vi "MAIN.vi"() -> ()   [LabVIEW 2015]
uses:
  <vilib>/addons/database/Connection.llb/Conn ObjectReference.ctl
  <vilib>/Utility/miscctls.llb/LVPointTypeDef.ctl
  <vilib>/Utility/file.llb/Read Delimited Spreadsheet (string).vi
  <vilib>/addons/database/Connection.llb/DB Tools Open Connec (Path).vi
  <vilib>/Utility/file.llb/Write Delimited Spreadsheet (string).vi
  <vilib>/addons/database/NI_Database_API.lvlib
panel:
  in  "MATOME":string
  out "userInfo":T1
  out "Connection Database":bool
  out "connection reference":T2
  out "info database":T3
  in  "Update to Database":bool
  out "size(s) 2":i32
  out "size(s)":i32
  out "Status":string
  out "LOT 2":string
  out "LOT 1":string
  out "mau array":string[][](array[string])
  in  "Create file program":bool
  out "sw array":string[][](array[string])
  out "matrix array":string[][](array[string])
  out "ong2 array":string[][](array[string])
  out "ong1 array":string[][](array[string])
  out "jigu array":string[][](array[string])
  in  "File Path Control":path caption="Load File"
  in  "STEP":string
  in  "REV":string
  in  "MODEL":string
  in  "Stop Button":bool
  in  "Save file":bool
  in  "Table Control":string[][](table)
  # "WRITE PROGRAM FOR CONTROL BOX MATOME"
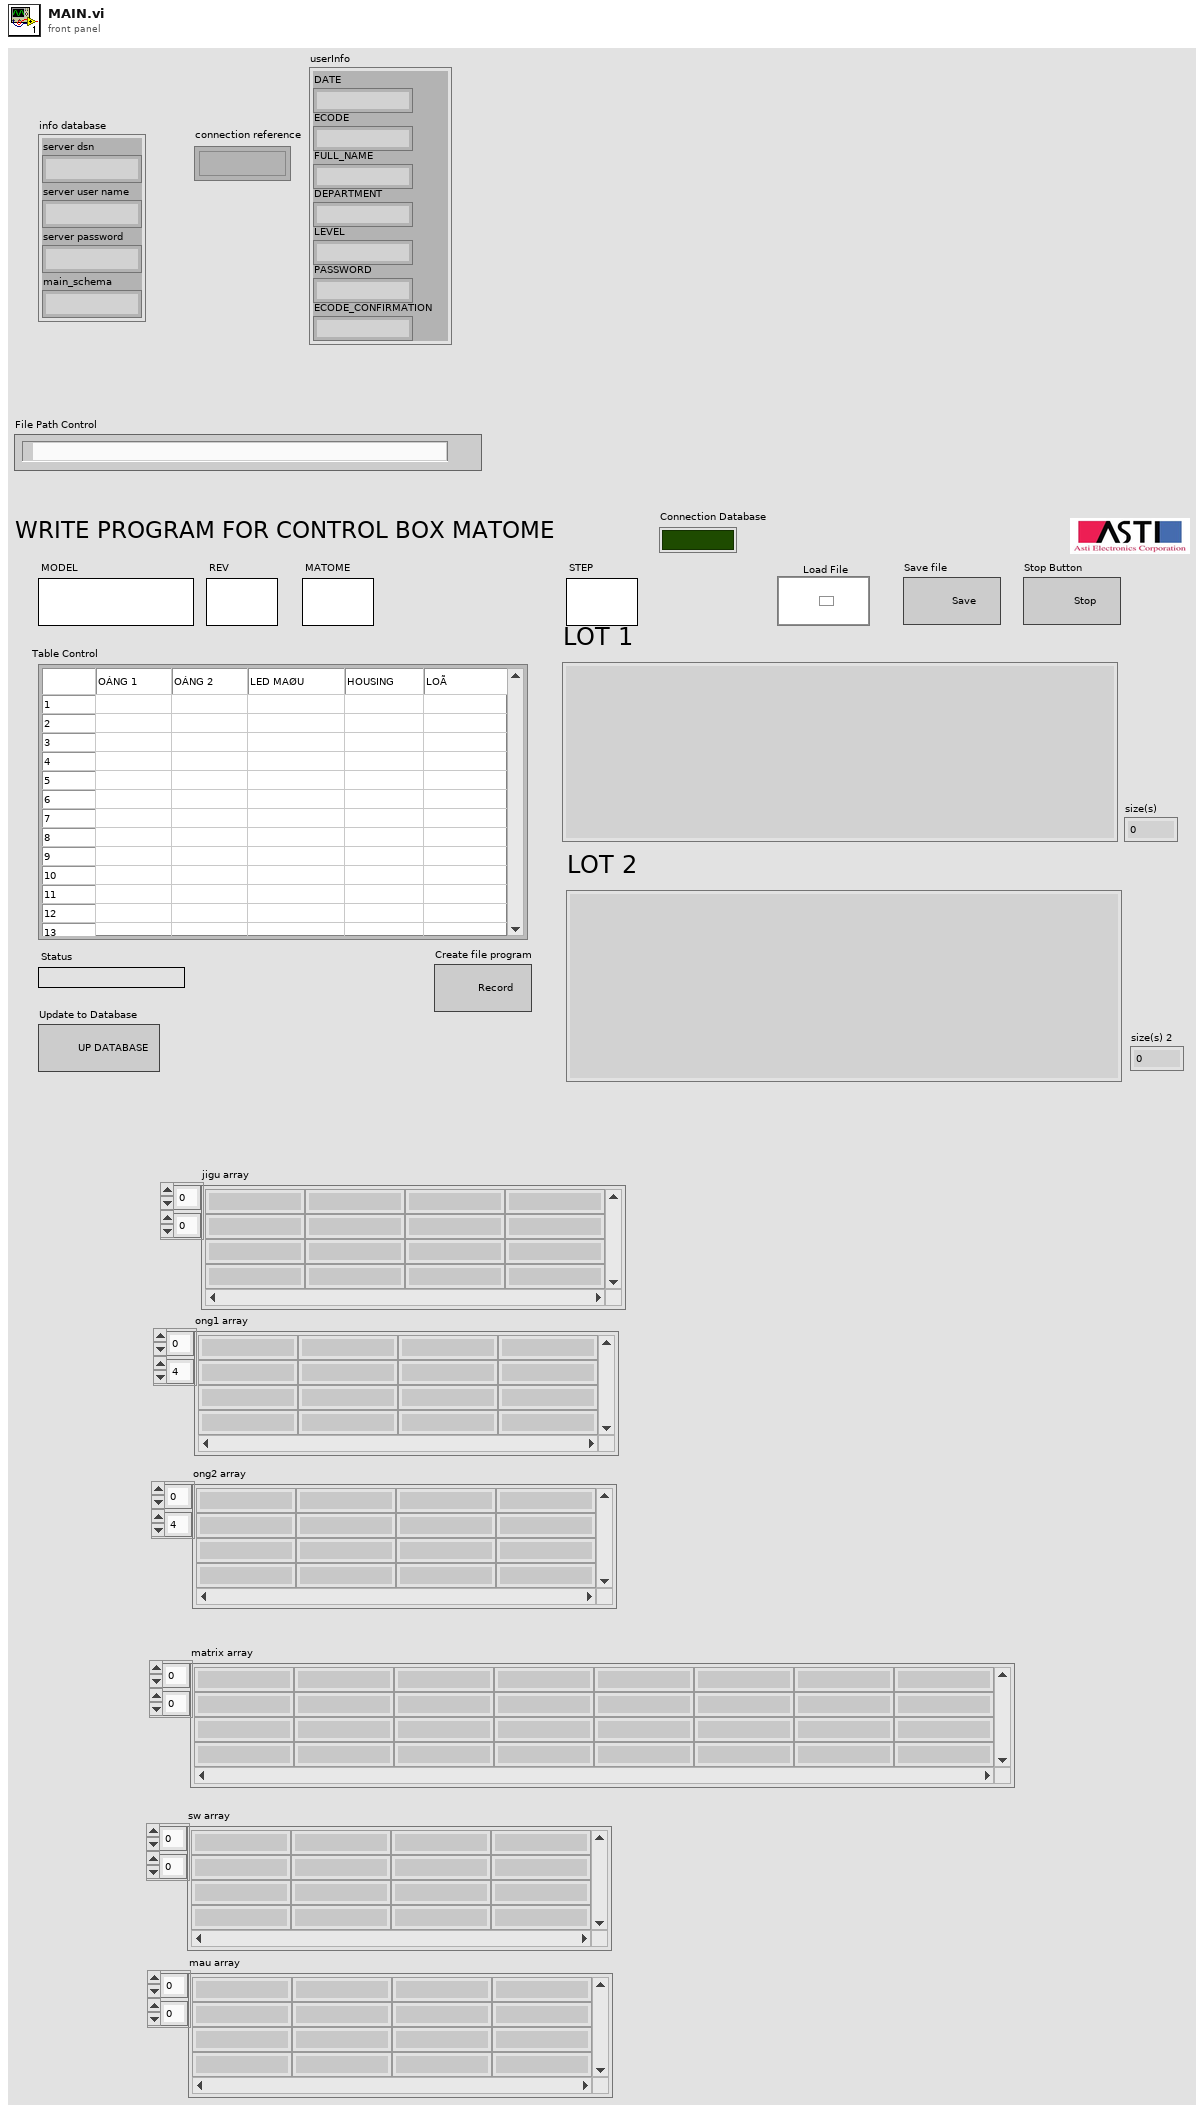
[diagram p1: front panel]
types:
  T1 = cluster{"DATE":string, "ECODE":string, "FULL_NAME":string, "DEPARTMENT":string, "LEVEL":string, "PASSWORD":string, "ECODE_CONFIRMATION":string}
  T2 = typedef "NI_Database_API.lvlib/Conn ObjectReference.ctl" = refnum<k1>
  T3 = cluster{"server dsn":string, "server user name":string, "server password":string, "main_schema":string}
  T4 = typedef "LVPointTypeDef.ctl" = cluster{"Horizontal":i16, "Vertical":i16}
  T5 = cluster{"date/time string":string, "LOT 1":string, "LOT 2":string, "ECODE":string}
  T6 = cluster{"date/time string":string, "MODEL":string, "REV":string, "LOT 1":string, "LOT 2":string, "ECODE":string, "MATOME":string}
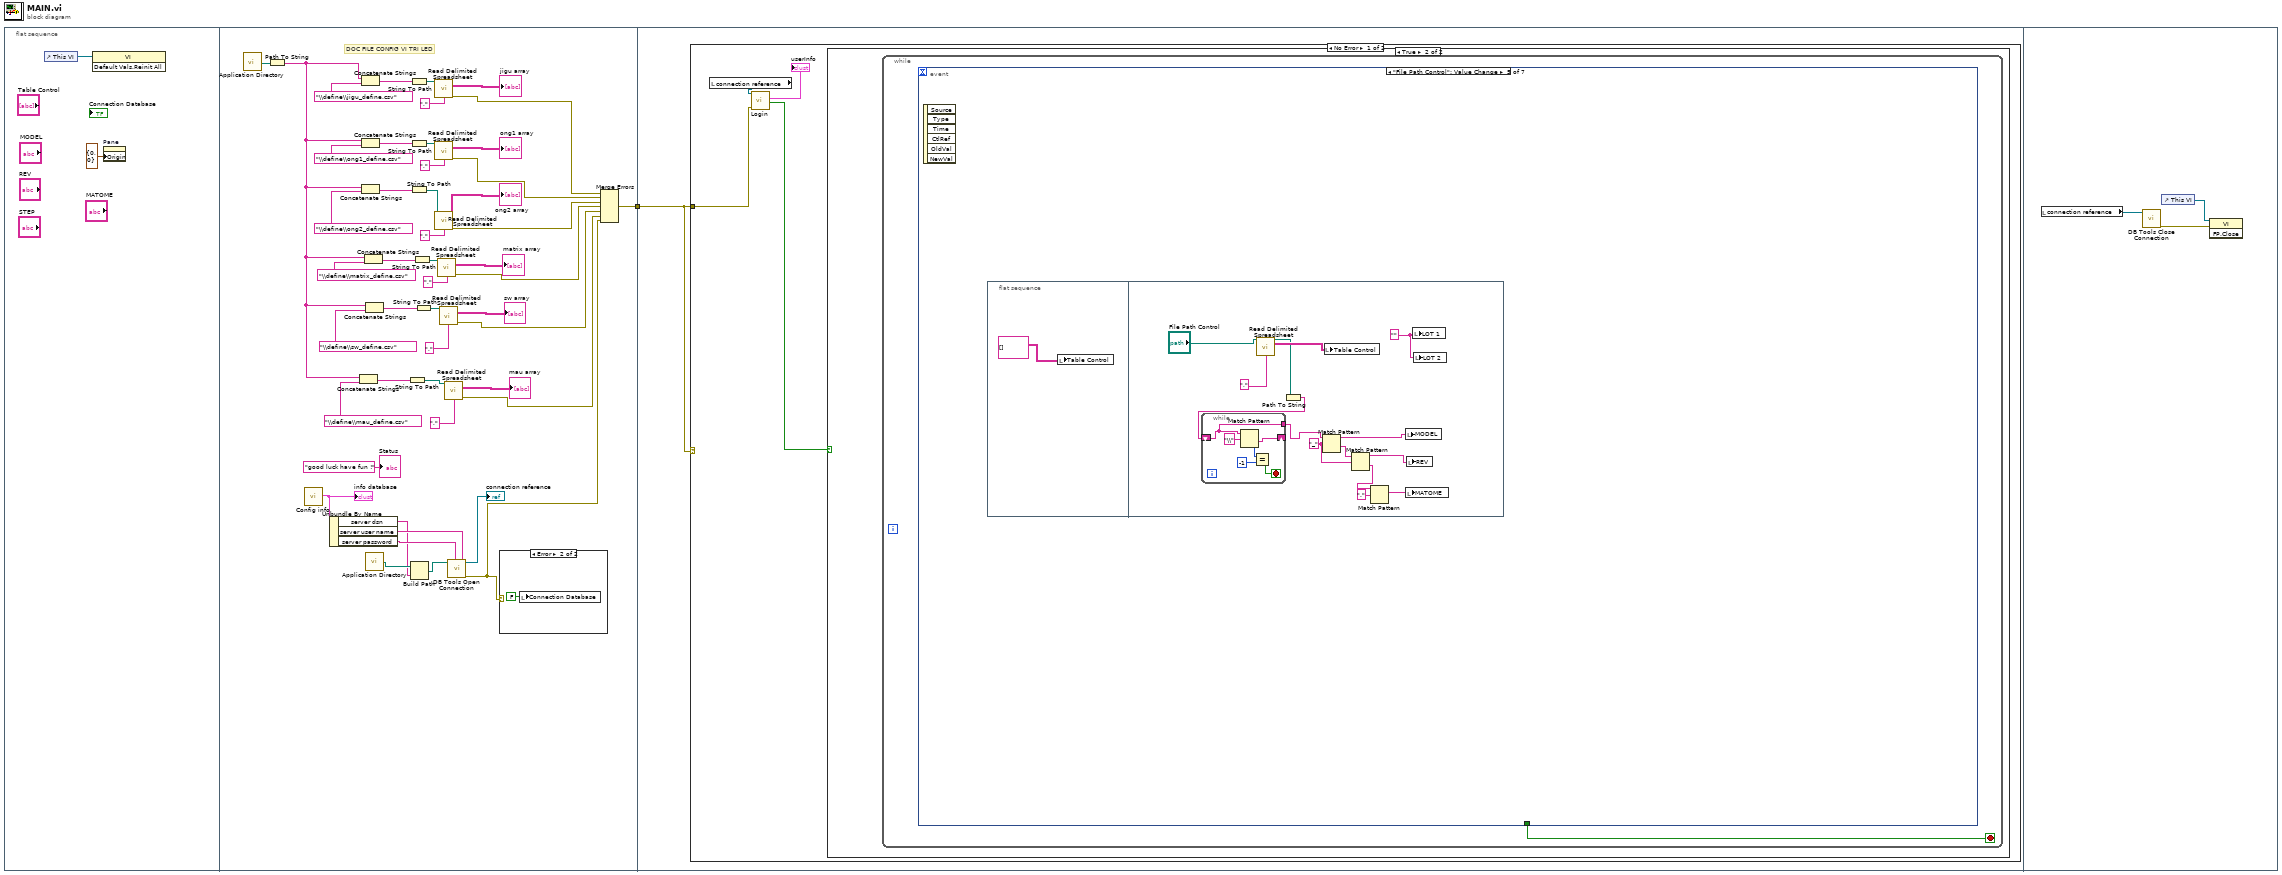
[diagram p0: block diagram]
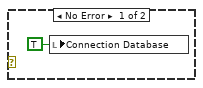
[diagram p2: hidden frame]
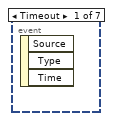
[diagram p4: hidden frame]
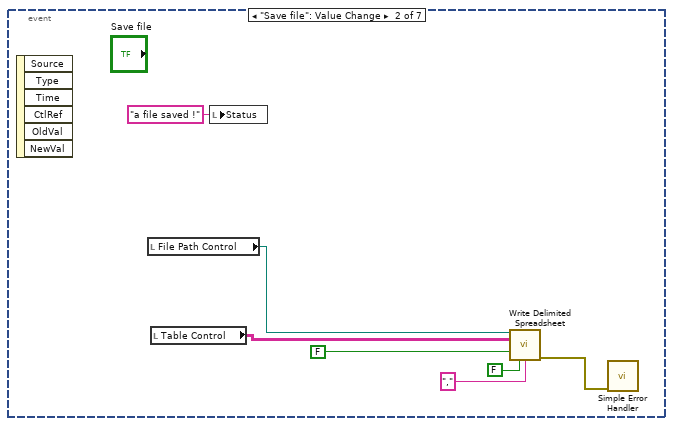
[diagram p5: hidden frame]
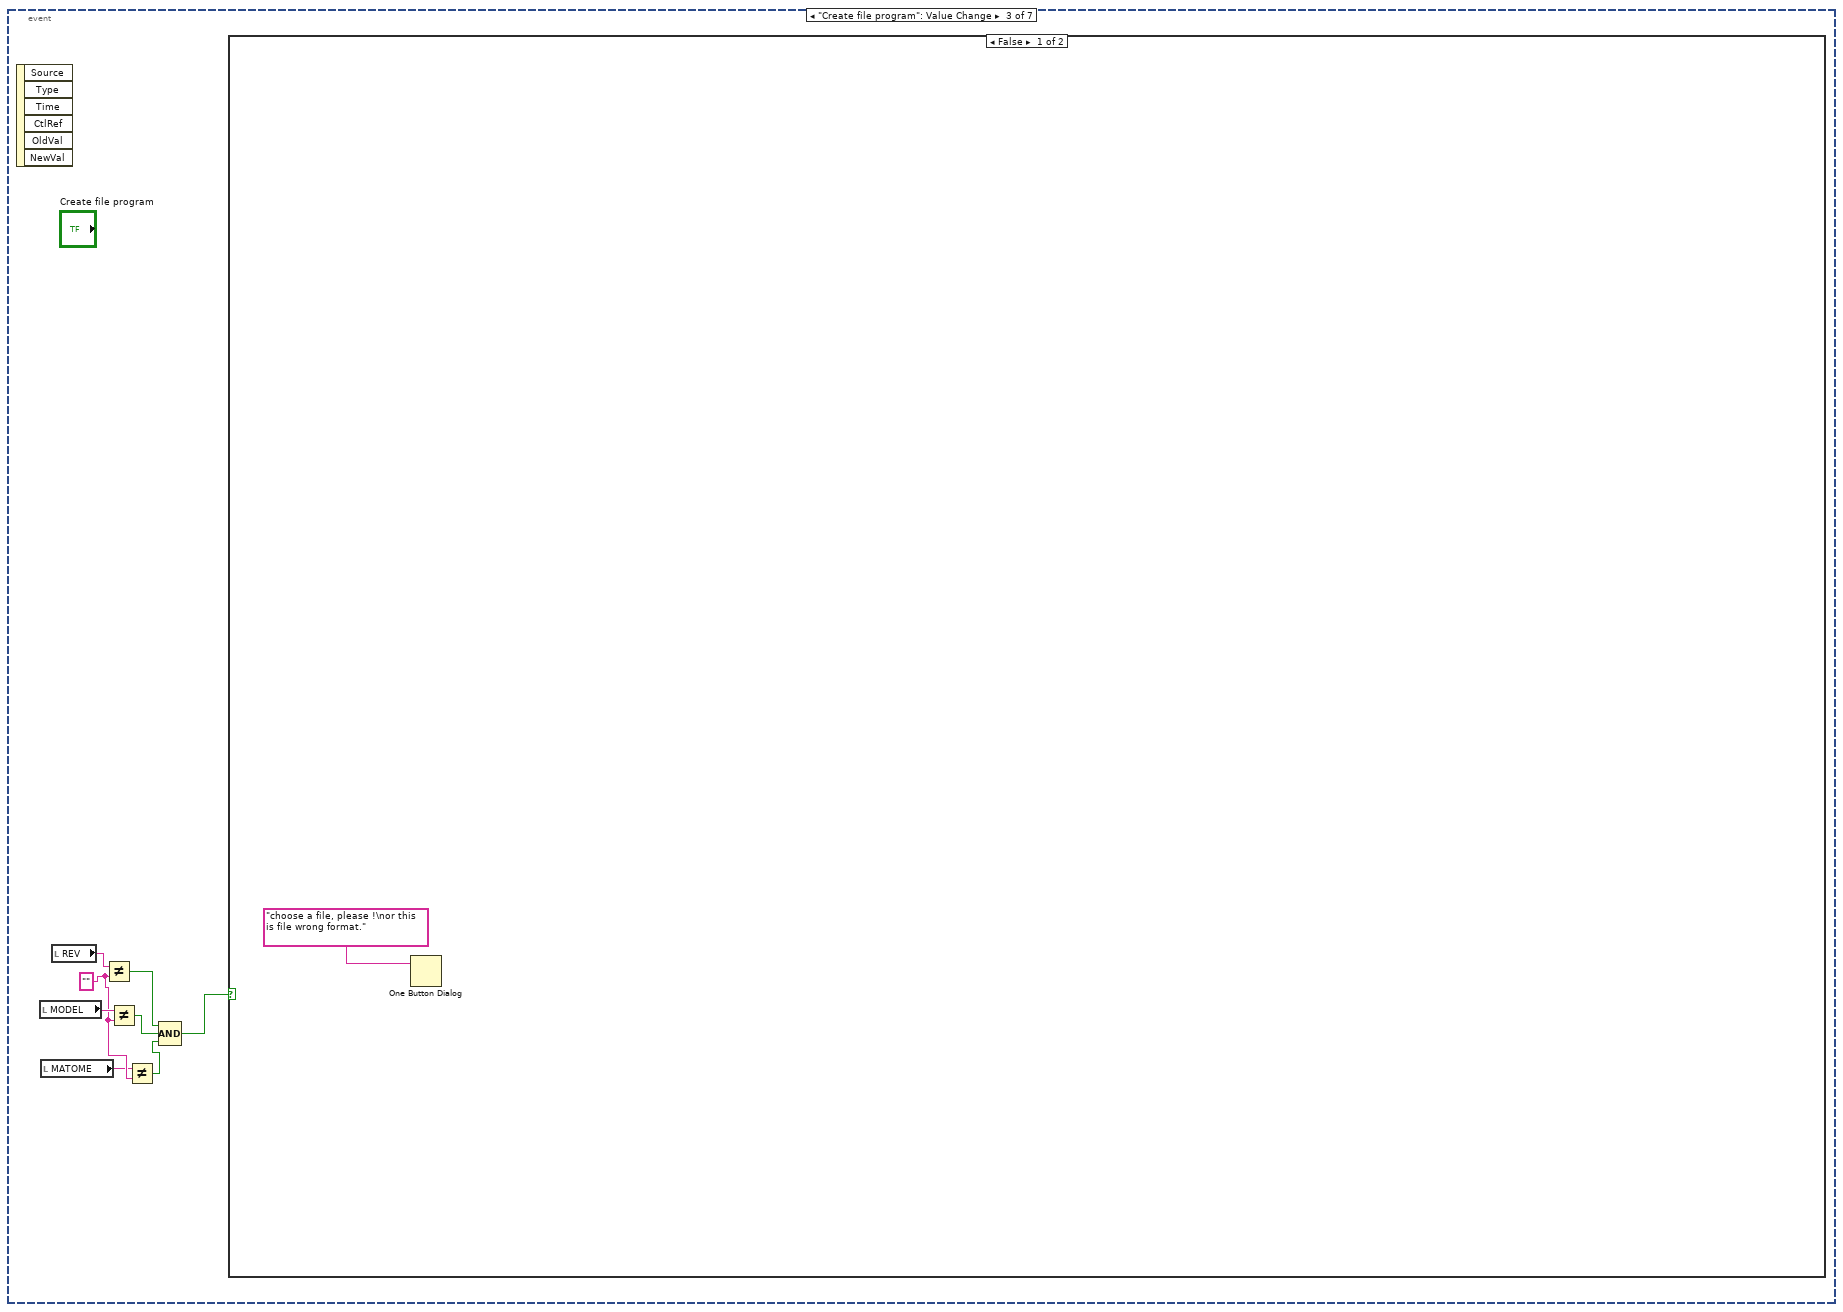
[diagram p6: hidden frame]
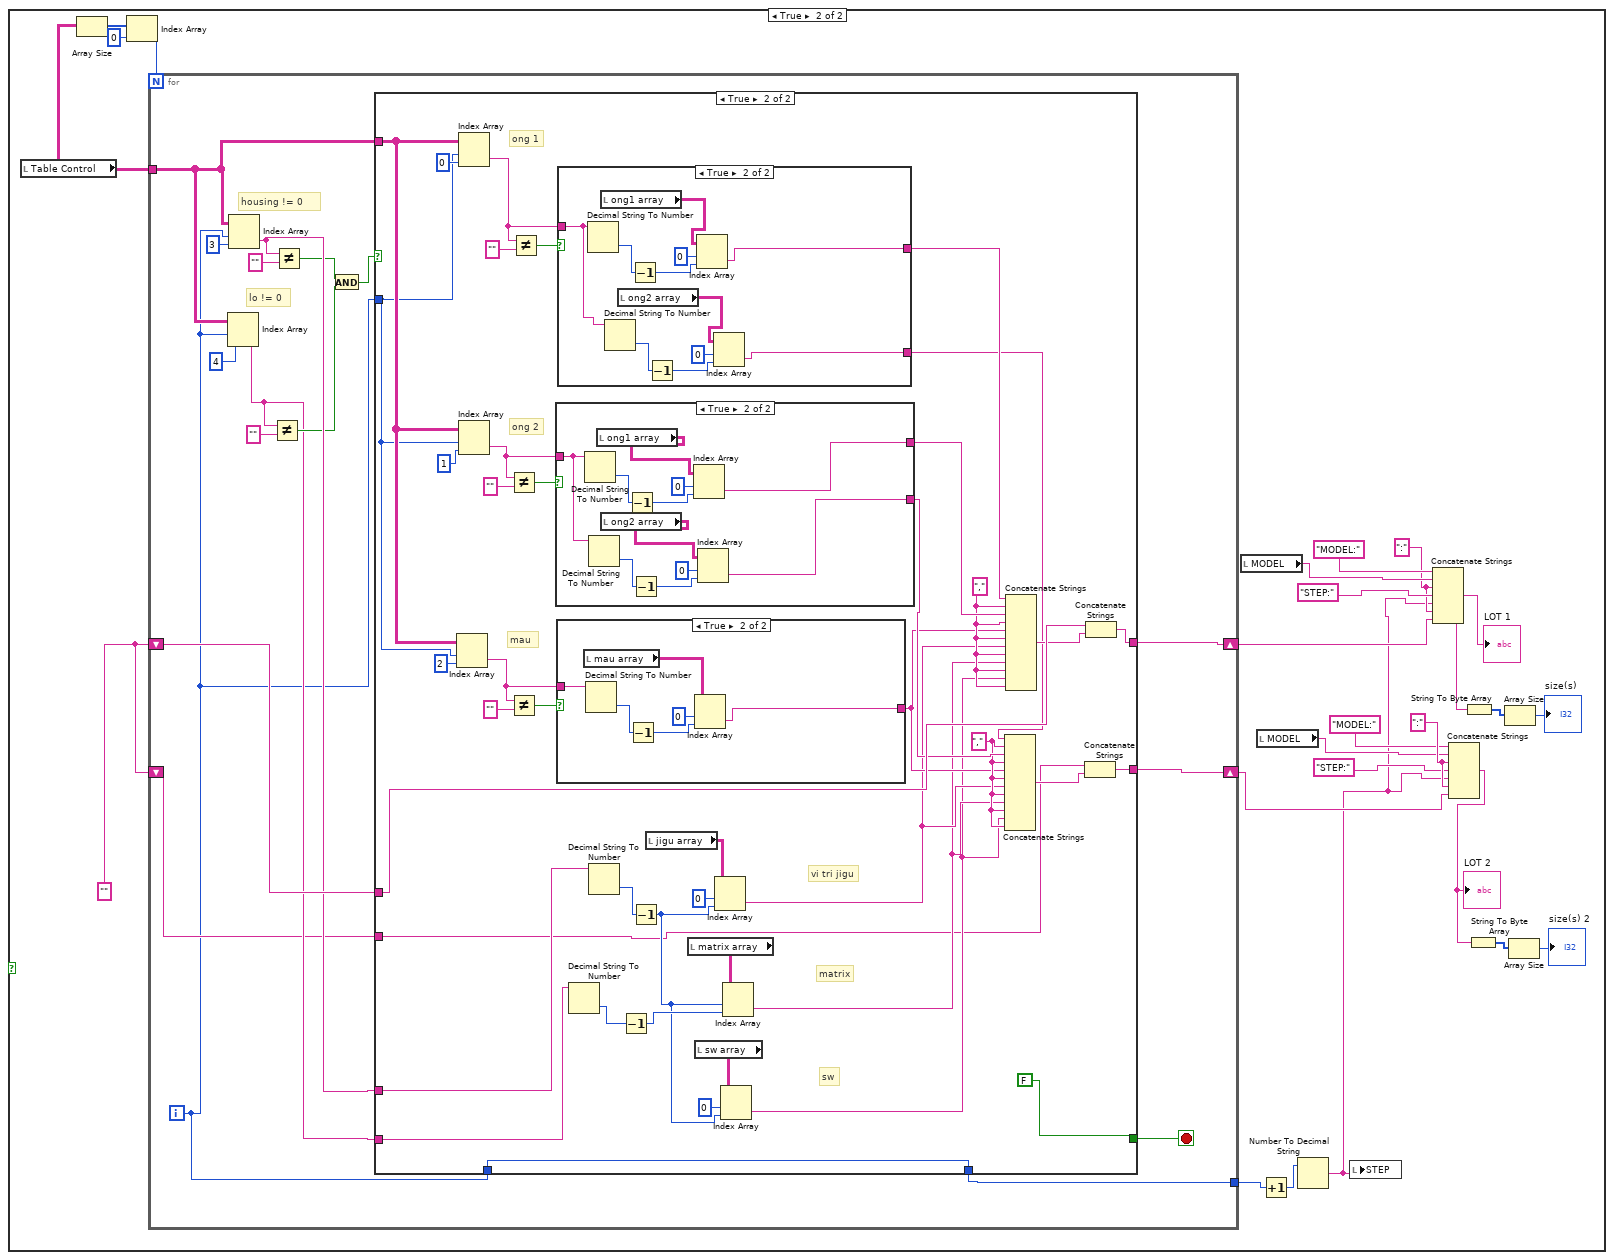
[diagram p7: hidden frame]
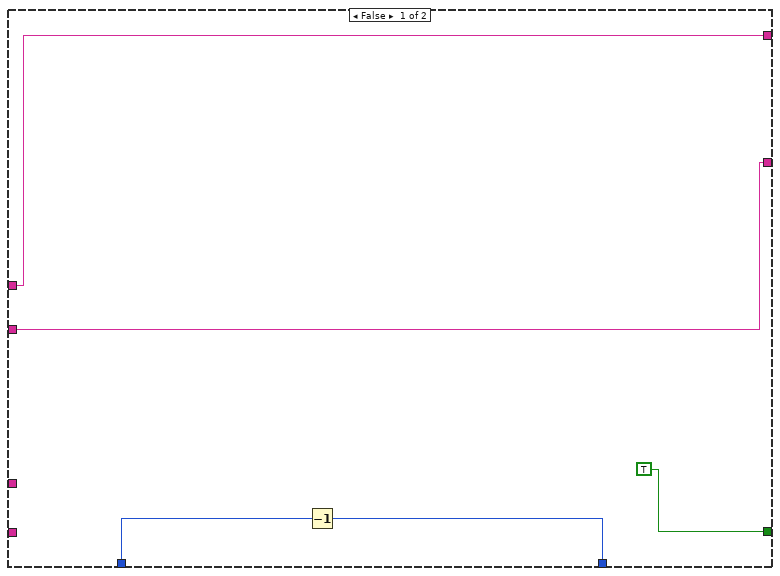
[diagram p8: hidden frame]
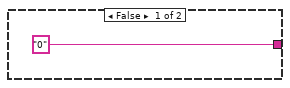
[diagram p9: hidden frame]
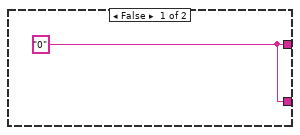
[diagram p10: hidden frame]
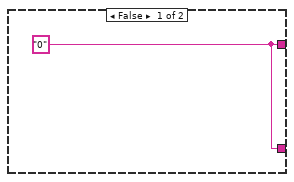
[diagram p11: hidden frame]
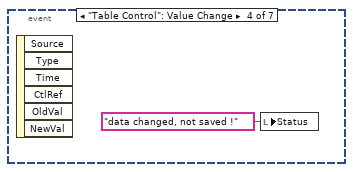
[diagram p12: hidden frame]
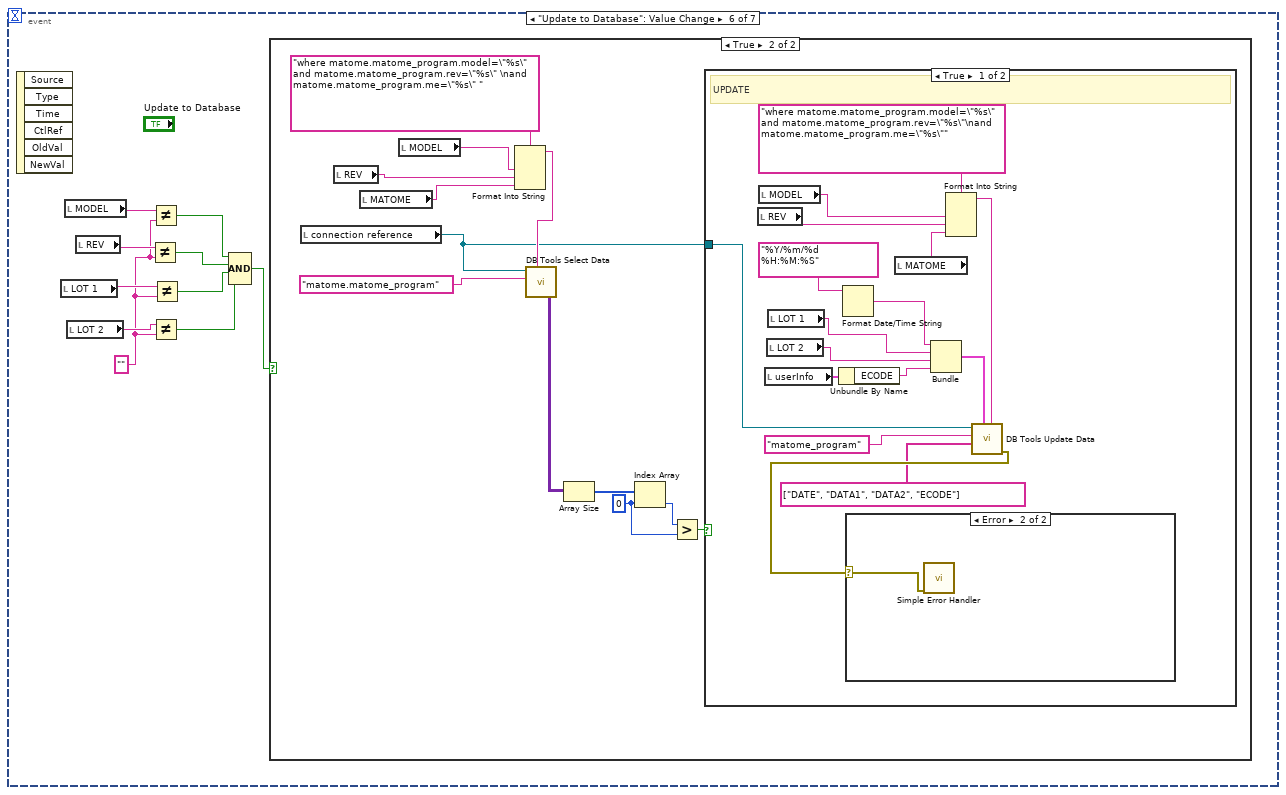
[diagram p13: hidden frame]
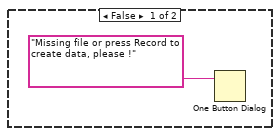
[diagram p14: hidden frame]
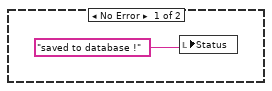
[diagram p15: hidden frame]
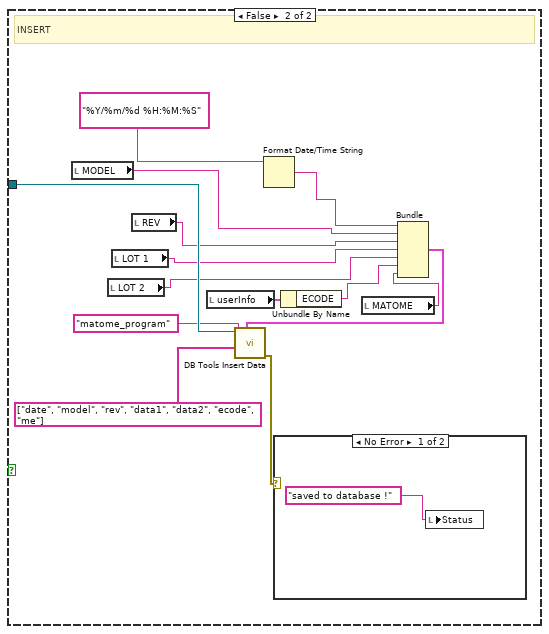
[diagram p16: hidden frame]
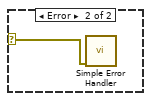
[diagram p17: hidden frame]
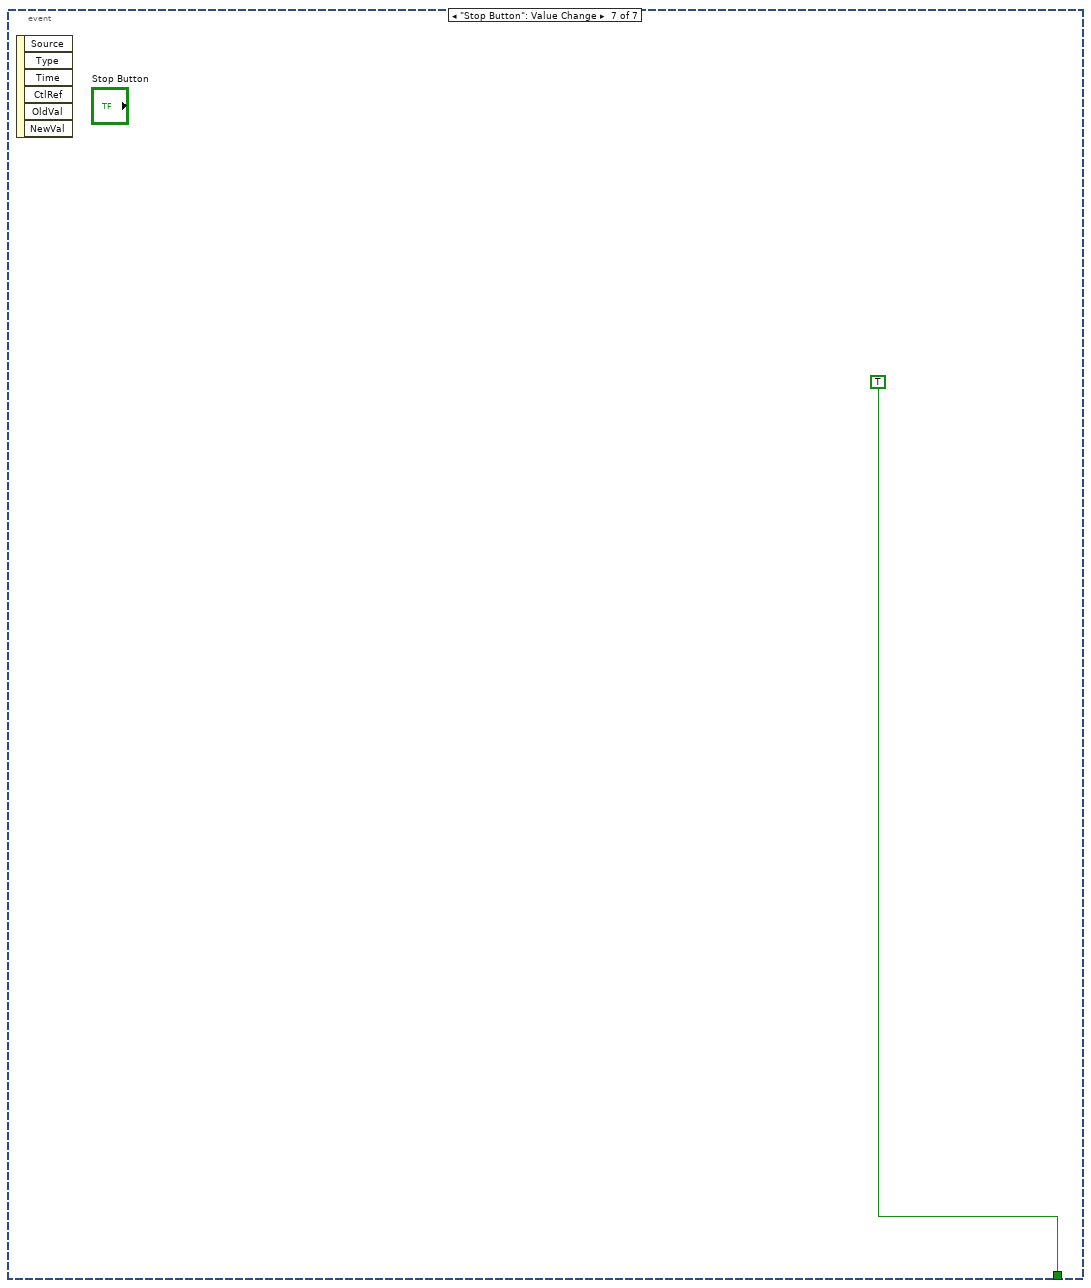
[diagram p18: hidden frame]
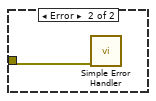
[diagram p19: hidden frame]
diagram:
  n1 = flat-sequence {
    tunnel: [w4] -> w1
    tunnel: w1 -> [w54]
    frame #0 {
      n2 = control-ref of="This VI"() -> (w3:refnum<vi>)
      n3 = invoke class="VI" method="Default Vals.Reinit All"(reference=w3) -> ()  [unwired: 2 in, 3 out]
      n4 = property on="Pane" class="Pane"("Origin"=T4 {"Horizontal"=0, "Vertical"=0}) -> ()  [unwired: 2 in, 2 out]
    }
    frame #1 {
      # "DOC FILE CONFIG VI TRI LED"
      n5 = call <vilib>:"Application Directory.vi"() -> ("Application Directory"=w51:path)
      n6 = Path To String(path=w51) -> (string=w20:string)
      n7 = call "Config info.vi"() -> ("info database"=w18:T3)  [unwired: 10 in, 1 out]
      "info database" <- w18
      n8 = Unbundle By Name(w18) -> ("server dsn"=w14:string, "server user name"=w17:string, "server password"=w16:string)
      n9 = Concatenate Strings(w20, "\\define\\mau_define.csv" ("string")) -> (w22:string)
      n10 = Concatenate Strings(w20, "\\define\\jigu_define.csv" ("string")) -> (w49:string)
      n11 = Concatenate Strings(w20, "\\define\\ong1_define.csv" ("string")) -> (w42:string)
      n12 = Concatenate Strings(w20, "\\define\\ong2_define.csv" ("string")) -> (w39:string)
      n13 = Concatenate Strings(w20, "\\define\\matrix_define.csv" ("string")) -> (w32:string)
      n14 = Concatenate Strings(w20, "\\define\\sw_define.csv" ("string")) -> (w29:string)
      n15 = call <vilib>:"Application Directory.vi"() -> ("Application Directory"=w15:path)
      n16 = String To Path(string=w22) -> (path=w23:path)
      n17 = Build Path(base path=w15, name or relative path=w14) -> (appended path=w13:path)
      n18 = String To Path(string=w49) -> (path=w48:path)
      n19 = String To Path(string=w42) -> (path=w43:path)
      n20 = String To Path(string=w39) -> (path=w38:path)
      n21 = String To Path(string=w32) -> (path=w33:path)
      n22 = String To Path(string=w29) -> (path=w28:path)
      n23 = call-poly <vilib>:"Read Delimited Spreadsheet.vi"("file path (dialog if empty)"=w48, "delimiter (\\t)"="," ("delimiter (\\t)")) -> ("all rows"=→"jigu array":string[][], "error out"=w11:errorcluster)  [unwired: 8 in, 4 out]
      n24 = call-poly <vilib>:"Read Delimited Spreadsheet.vi"("file path (dialog if empty)"=w43, "delimiter (\\t)"="," ("delimiter (\\t)")) -> ("all rows"=→"ong1 array":string[][], "error out"=w10:errorcluster)  [unwired: 8 in, 4 out]
      n25 = call-poly <vilib>:"Read Delimited Spreadsheet.vi"("file path (dialog if empty)"=w38, "delimiter (\\t)"="," ("delimiter (\\t)")) -> ("all rows"=→"ong2 array":string[][], "error out"=w9:errorcluster)  [unwired: 8 in, 4 out]
      n26 = call-poly <vilib>:"Read Delimited Spreadsheet.vi"("file path (dialog if empty)"=w33, "delimiter (\\t)"="," ("delimiter (\\t)")) -> ("all rows"=→"matrix array":string[][], "error out"=w8:errorcluster)  [unwired: 8 in, 4 out]
      n27 = call-poly <vilib>:"Read Delimited Spreadsheet.vi"("file path (dialog if empty)"=w28, "delimiter (\\t)"="," ("delimiter (\\t)")) -> ("all rows"=→"sw array":string[][], "error out"=w7:errorcluster)  [unwired: 8 in, 4 out]
      n28 = call-poly <vilib>:"Read Delimited Spreadsheet.vi"("file path (dialog if empty)"=w23, "delimiter (\\t)"="," ("delimiter (\\t)")) -> ("all rows"=→"mau array":string[][], "error out"=w6:errorcluster)  [unwired: 8 in, 4 out]
      n29 = call-poly <vilib>:"DB Tools Open Connection.vi"("password"=w16, "userID"=w17, "connection information"=w13) -> ("error out"=w5:errorcluster, "connection reference"=→"connection reference":T2)  [unwired: 5 in]
      n30 = case shown="Error" w5 {
        frame No Error {
          n31 = local write "Connection Database"(TRUE ("Connection Database")) -> ()
        }
        frame Error {
          n32 = local write "Connection Database"(FALSE ("Connection Database")) -> ()
        }
      }
      n33 = Merge Errors(w11, w10, w9, w8, w7, w6, w5) -> (w4:errorcluster)
      "Status" <- "good luck have fun !" ("Status")
    }
    frame #2 {
      n34 = case shown="No Error" w54 {
        tunnel: w54 -> [w55 w276]
        frame No Error {
          n35 = local read "connection reference"() -> (w58:T2)
          n36 = call "Login.vi"("error in (no error)"=w55, "connection reference"=w58) -> ("valid?"=w57:bool, "userInfo"=→"userInfo":T1)  [unwired: 6 in, 2 out]
          n37 = case shown="True" w57 {
            frame False {
            }
            frame True {
              n38 = while {
                stop <- w59 stop-if-true
                n39 = event shown="[4] \"File Path Control\": Value Change" {
                  selector: _ -> [_ _ _ _ _ _ _]
                  dyn-events: _ -> [_ _ _ _ _ _ _]
                  timeout: _ -> [_ _ _ _ _ _ _]
                  tunnel: [_ _ _ _ _ _ TRUE] -> w59
                  event Timeout {
                    n40 = event-data() -> ()  [unwired: 1 in, 3 out]
                  }
                  event "Save file": Value Change {
                    n41 = event-data() -> ()  [unwired: 1 in, 6 out]
                    n42 = local read "File Path Control"() -> (w66:path)
                    n43 = local read "Table Control"() -> (w65:string[][])
                    n44 = local write "Status"("a file saved !" ("Status")) -> ()
                    n45 = call-poly <vilib>:"Write Delimited Spreadsheet.vi"("file path (dialog if empty)"=w66, "2D data"=w65, "append to file? (F)"=FALSE, "transpose? (F)"=FALSE, "delimiter (\\t)"="," ("delimiter (\\t)")) -> ("error out"=w61:errorcluster)  [unwired: 9 in, 1 out]
                    n46 = call <vilib>:"Simple Error Handler.vi"("error in (no error)"=w61) -> ()  [unwired: 4 in, 5 out]
                  }
                  event "Create file program": Value Change {
                    w72 = ""
                    n47 = event-data() -> ()  [unwired: 1 in, 6 out]
                    n48 = local read "MODEL"() -> (w73:string)
                    n49 = local read "MATOME"() -> (w71:string)
                    n50 = local read "REV"() -> (w74:string)
                    n51 = Not Equal?(x=w74, y=w72) -> (x != y?=w70:bool)
                    n52 = Not Equal?(x=w73, y=w72) -> (x != y?=w69:bool)
                    n53 = Not Equal?(x=w71, y=w72) -> (x != y?=w68:bool)
                    n54 = Compound Arithmetic op=AND(w70, w69, w68) -> (w67:bool)
                    n55 = case shown="False" w67 {
                      frame False {
                        n56 = One Button Dialog(message="choose a file, please !\nor this is file wrong format.") -> ()  [unwired: 1 in, 1 out]
                      }
                      frame True {
                        w89 = ":" ("string")
                        w91 = ":" ("string")
                        w95 = ""
                        n57 = local read "Table Control"() -> (w96:string[][])
                        n58 = Array Size(array=w96) -> (size(s)=w99:i32[])
                        n59 = Index Array(array=w99, index=0) -> (element=w97:i32)
                        n60 = for {
                          N: w97 -> [_]
                          tunnel: w96 -> [w110]
                          shift-right: [w105] -> w90
                          shift-left: w95 -> [w114]
                          shift-right: [w103] -> w86
                          shift-left: w95 -> [w102]
                          tunnel: [w100] -> w84
                          i -> [w101]
                          stop <- w104 stop-if-true
                          # "lo != 0"
                          # "housing != 0"
                          n61 = Index Array(array=w110, index (row)=w101, index (col)=4 ("disabled index (col)")) -> (element=w106:string)
                          n62 = Index Array(array=w110, index (row)=w101, index (col)=3 ("disabled index (col)")) -> (element=w113:string)
                          n63 = Not Equal?(x=w106, y="") -> (x != y?=w108:bool)
                          n64 = Not Equal?(x=w113, y="") -> (x != y?=w109:bool)
                          n65 = And(x=w109, y=w108) -> (x .and. y?=w107:bool)
                          n66 = case shown="True" w107 {
                            tunnel: w114 -> [w121 w136]
                            tunnel: w110 -> [_ w152]
                            tunnel: w101 -> [_ w151]
                            tunnel: w113 -> [_ w147]
                            tunnel: w106 -> [_ w145]
                            tunnel: [w121 w134] -> w105
                            tunnel: [TRUE FALSE] -> w104
                            tunnel: [w119 w124] -> w103
                            tunnel: w102 -> [w119 w123]
                            tunnel: w101 -> [w118 w122]
                            tunnel: [w117 w122] -> w100
                            frame False {
                              n67 = Decrement(x=w118) -> (x-1=w117:i32)
                            }
                            frame True {
                              w129 = ","
                              w137 = ","
                              # "sw"
                              # "matrix"
                              # "vi tri jigu"
                              # "mau"
                              # "ong 2"
                              # "ong 1"
                              n68 = Index Array(array=w152, index (row)=w151, index (col)=2 ("disabled index (col)")) -> (element=w153:string)
                              n69 = Index Array(array=w152, index (row)=w151, index (col)=0 ("disabled index (col)")) -> (element=w161:string)
                              n70 = Index Array(array=w152, index (row)=w151, index (col)=1 ("disabled index (col)")) -> (element=w160:string)
                              n71 = Not Equal?(x=w160, y="") -> (x != y?=w159:bool)
                              n72 = Not Equal?(x=w153, y="") -> (x != y?=w154:bool)
                              n73 = Not Equal?(x=w161, y="") -> (x != y?=w162:bool)
                              n74 = case shown="True" w159 {
                                tunnel: [w172 w180] -> w138
                                tunnel: w160 -> [_ w174]
                                tunnel: [w172 w173] -> w130
                                frame False {
                                w172 = "0"
                                }
                                frame True {
                                n75 = Decimal String To Number(string=w174) -> (number=w182:i32)  [unwired: 2 in, 1 out]
                                n76 = Decimal String To Number(string=w174) -> (number=w176:i32)  [unwired: 2 in, 1 out]
                                n77 = local read "ong1 array"() -> (w179:string[][])
                                n78 = local read "ong2 array"() -> (w178:string[][])
                                n79 = Decrement(x=w182) -> (x-1=w181:i32)
                                n80 = Decrement(x=w176) -> (x-1=w177:i32)
                                n81 = Index Array(array=w179, index (row)=0, index (col)=w181) -> (element=w180:string)
                                n82 = Index Array(array=w178, index (row)=0, index (col)=w177) -> (element=w173:string)
                                }
                              }
                              n83 = case shown="True" w154 {
                                tunnel: ["0" w166] -> w128
                                tunnel: w153 -> [_ w169]
                                frame False {
                                }
                                frame True {
                                n84 = local read "mau array"() -> (w171:string[][])
                                n85 = Decimal String To Number(string=w169) -> (number=w168:i32)  [unwired: 2 in, 1 out]
                                n86 = Decrement(x=w168) -> (x-1=w167:i32)
                                n87 = Index Array(array=w171, index (row)=0, index (col)=w167) -> (element=w166:string)
                                }
                              }
                              n88 = case shown="True" w162 {
                                tunnel: [w184 w192] -> w139
                                tunnel: w161 -> [_ w186]
                                tunnel: [w184 w185] -> w131
                                frame False {
                                w184 = "0"
                                }
                                frame True {
                                n89 = Decimal String To Number(string=w186) -> (number=w194:i32)  [unwired: 2 in, 1 out]
                                n90 = local read "ong1 array"() -> (w191:string[][])
                                n91 = Decimal String To Number(string=w186) -> (number=w188:i32)  [unwired: 2 in, 1 out]
                                n92 = local read "ong2 array"() -> (w190:string[][])
                                n93 = Decrement(x=w194) -> (x-1=w193:i32)
                                n94 = Decrement(x=w188) -> (x-1=w189:i32)
                                n95 = Index Array(array=w191, index (row)=0, index (col)=w193) -> (element=w192:string)
                                n96 = Index Array(array=w190, index (row)=0, index (col)=w189) -> (element=w185:string)
                                }
                              }
                              n97 = Decimal String To Number(string=w145) -> (number=w144:i32)  [unwired: 2 in, 1 out]
                              n98 = Decimal String To Number(string=w147) -> (number=w148:i32)  [unwired: 2 in, 1 out]
                              n99 = Decrement(x=w144) -> (x-1=w143:i32)
                              n100 = Decrement(x=w148) -> (x-1=w141:i32)
                              n101 = local read "jigu array"() -> (w150:string[][])
                              n102 = local read "matrix array"() -> (w146:string[][])
                              n103 = local read "sw array"() -> (w142:string[][])
                              n104 = Index Array(array=w150, index (row)=0, index (col)=w141) -> (element=w127:string)
                              n105 = Index Array(array=w142, index (row)=0 ("disabled index (row)"), index (col)=w141) -> (element=w125:string)
                              n106 = Index Array(array=w146, index (row)=w141, index (col)=w143) -> (element=w126:string)
                              n107 = Concatenate Strings(w131, w129, w130, w129, w128, w129, w127, w129, w126, w129, w125, w129) -> (w132:string)
                              n108 = Concatenate Strings(w139, w137, w138, w137, w128, w137, w127, w137, w126, w137, w125, w137) -> (w135:string)
                              n109 = Concatenate Strings(w123, w132) -> (w124:string)
                              n110 = Concatenate Strings(w136, w135) -> (w134:string)
                            }
                          }
                        }
                        n111 = local read "MODEL"() -> (w93:string)
                        n112 = local read "MODEL"() -> (w88:string)
                        n113 = Increment(x=w84) -> (x+1=w85:i32)
                        n114 = Number To Decimal String(number=w85) -> (decimal integer string=w82:string)  [unwired: 1 in]
                        n115 = local write "STEP"(w82) -> ()
                        n116 = Concatenate Strings("MODEL:" ("string"), w93, w91, "STEP:" ("string"), w82, w91, w90) -> (w81:string)
                        "LOT 1" <- w81
                        n117 = Concatenate Strings("MODEL:" ("string"), w88, w89, "STEP:" ("string"), w82, w89, w86) -> (w76:string)
                        "LOT 2" <- w76
                        n118 = String To Byte Array(string=w81) -> (unsigned byte array=w80:u8[])
                        n119 = String To Byte Array(string=w76) -> (unsigned byte array=w77:u8[])
                        n120 = Array Size(array=w80) -> (size(s)=→"size(s)":i32)
                        n121 = Array Size(array=w77) -> (size(s)=→"size(s) 2":i32)
                      }
                    }
                  }
                  event "Table Control": Value Change {
                    n122 = event-data() -> ()  [unwired: 1 in, 6 out]
                    n123 = local write "Status"("data changed, not saved !" ("Status")) -> ()
                  }
                  event "File Path Control": Value Change {
                    n124 = event-data() -> ()  [unwired: 1 in, 6 out]
                    n125 = flat-sequence {
                      frame #0 {
                        n126 = local write "Table Control"(string[][] []) -> ()
                      }
                      frame #1 {
                        w198 = ""
                        w202 = "_" ("regular expression")
                        n127 = call-poly <vilib>:"Read Delimited Spreadsheet.vi"("file path (dialog if empty)"="File Path Control", "delimiter (\\t)"="," ("delimiter (\\t)")) -> ("new file path (Not A Path if cancelled)"=w208:path, "all rows"=w209:string[][])  [unwired: 8 in, 4 out]
                        n128 = Path To String(path=w208) -> (string=w207:string)
                        n129 = while {
                          shift-right: [w213] -> _
                          shift-left: w207 -> [w212]
                          tunnel: [w212] -> w206
                          stop <- w214 stop-if-true
                          n130 = Match Pattern(string=w212, regular expression="\\") -> (after substring=w213:string, offset past match=w216:i32)  [unwired: 1 in, 2 out]
                          n131 = Equal?(x=w216, y=-1) -> (x = y?=w214:bool)
                        }
                        n132 = Match Pattern(string=w206, regular expression=w202) -> (before substring=w205:string, after substring=w203:string)  [unwired: 1 in, 2 out]
                        n133 = local write "Table Control"(w209) -> ()
                        n134 = Match Pattern(string=w203, regular expression=w202) -> (before substring=w200:string, after substring=w201:string)  [unwired: 1 in, 2 out]
                        n135 = Match Pattern(string=w201, regular expression=".") -> (match substring=w199:string)  [unwired: 1 in, 3 out]
                        n136 = local write "MODEL"(w205) -> ()
                        n137 = local write "MATOME"(w199) -> ()
                        n138 = local write "REV"(w200) -> ()
                        n139 = local write "LOT 1"(w198) -> ()
                        n140 = local write "LOT 2"(w198) -> ()
                      }
                    }
                  }
                  event "Update to Database": Value Change {
                    w223 = ""
                    n141 = event-data() -> ()  [unwired: 1 in, 6 out]
                    n142 = local read "LOT 1"() -> (w225:string)
                    n143 = local read "MODEL"() -> (w227:string)
                    n144 = local read "LOT 2"() -> (w224:string)
                    n145 = local read "REV"() -> (w226:string)
                    n146 = Not Equal?(x=w226, y=w223) -> (x != y?=w221:bool)
                    n147 = Not Equal?(x=w227, y=w223) -> (x != y?=w222:bool)
                    n148 = Not Equal?(x=w224, y=w223) -> (x != y?=w219:bool)
                    n149 = Not Equal?(x=w225, y=w223) -> (x != y?=w220:bool)
                    n150 = Compound Arithmetic op=AND(w222, w221, w220, w219) -> (w218:bool)
                    n151 = case shown="True" w218 {
                      frame False {
                        n152 = One Button Dialog(message="Missing file or press Record to create data, please !") -> ()  [unwired: 1 in, 1 out]
                      }
                      frame True {
                        w236 = 0 ("index")
                        n153 = local read "connection reference"() -> (w231:T2)
                        n154 = local read "REV"() -> (w230:string)
                        n155 = local read "MATOME"() -> (w229:string)
                        n156 = local read "MODEL"() -> (w232:string)
                        n157 = Format Into String(format string="where matome.matome_program.model=\"%s\" and matome.matome_program.rev=\"%s\" \nand matome.matome_program.me=\"%s\" " ("condition"), w232, w230, w229) -> (resulting string=w233:string)  [unwired: 2 in, 1 out]
                        n158 = call <vilib>:"DB Tools Select Data.vi"("condition"=w233, "table"="matome.matome_program", "connection reference"=w231) -> ("data"=w239:variant[][])  [unwired: 3 in, 2 out]
                        n159 = Array Size(array=w239) -> (size(s)=w238:i32[])
                        n160 = Index Array(array=w238, index=w236) -> (element=w237:i32)
                        n161 = Greater?(x=w237, y=w236) -> (0:w235:bool)
                        n162 = case shown="True" w235 {
                          tunnel: w231 -> [w256 w272]
                          frame True {
                            # "UPDATE"
                            n163 = local read "REV"() -> (w251:string)
                            n164 = local read "MODEL"() -> (w252:string)
                            n165 = local read "userInfo"() -> (w245:T1)
                            n166 = local read "LOT 2"() -> (w246:string)
                            n167 = local read "LOT 1"() -> (w247:string)
                            n168 = Unbundle By Name(w245) -> ("ECODE"=w244:string)
                            n169 = Format Date/Time String(time format string (%c)="%Y/%m/%d %H:%M:%S") -> (date/time string=w248:string)  [unwired: 2 in]
                            n170 = local read "MATOME"() -> (w242:string)
                            n171 = Bundle("date/time string"=w248, "LOT 1"=w247, "LOT 2"=w246, "ECODE"=w244) -> (w250:T5)  [unwired: 1 in]
                            n172 = Format Into String(format string="where matome.matome_program.model=\"%s\" and matome.matome_program.rev=\"%s\"\nand matome.matome_program.me=\"%s\"", w252, w251, w242) -> (resulting string=w254:string)  [unwired: 2 in, 1 out]
                            n173 = call <vilib>:"DB Tools Update Data.vi"("condition"=w254, "data"=w250, "columns"=string[] ["DATE", "DATA1", "DATA2", "ECODE"], "table"="matome_program", "connection reference"=w256) -> ("error out"=w243:errorcluster)  [unwired: 5 in, 1 out]
                            n174 = case shown="Error" w243 {
                              selector: w243 -> [_ w258]
                              frame No Error {
                                n175 = local write "Status"("saved to database !" ("Status")) -> ()
                              }
                              frame Error {
                                n176 = call <vilib>:"Simple Error Handler.vi"("error in (no error)"=w258) -> ()  [unwired: 4 in, 5 out]
                              }
                            }
                          }
                          frame False {
                            # "INSERT"
                            n177 = local read "MODEL"() -> (w266:string)
                            n178 = local read "LOT 2"() -> (w263:string)
                            n179 = local read "LOT 1"() -> (w264:string)
                            n180 = local read "REV"() -> (w265:string)
                            n181 = local read "userInfo"() -> (w261:T1)
                            n182 = Format Date/Time String(time format string (%c)="%Y/%m/%d %H:%M:%S") -> (date/time string=w267:string)  [unwired: 2 in]
                            n183 = Unbundle By Name(w261) -> ("ECODE"=w260:string)
                            n184 = local read "MATOME"() -> (w259:string)
                            n185 = Bundle("date/time string"=w267, "MODEL"=w266, "REV"=w265, "LOT 1"=w264, "LOT 2"=w263, "ECODE"=w260, "MATOME"=w259) -> (w268:T6)  [unwired: 1 in]
                            n186 = call <vilib>:"DB Tools Insert Data.vi"("data"=w268, "columns"=string[] ["date", "model", "rev", "data1", "data2", "ecode", "me"], "table"="matome_program", "connection reference"=w272) -> ("error out"=w262:errorcluster)  [unwired: 6 in, 1 out]
                            n187 = case shown="No Error" w262 {
                              selector: w262 -> [_ w274]
                              frame No Error {
                                n188 = local write "Status"("saved to database !" ("Status")) -> ()
                              }
                              frame Error {
                                n189 = call <vilib>:"Simple Error Handler.vi"("error in (no error)"=w274) -> ()  [unwired: 4 in, 5 out]
                              }
                            }
                          }
                        }
                      }
                    }
                  }
                  event "Stop Button": Value Change {
                    n190 = event-data() -> ()  [unwired: 1 in, 6 out]
                  }
                }
              }
            }
          }
        }
        frame Error {
          n191 = call <vilib>:"Simple Error Handler.vi"("error in (no error)"=w276) -> ()  [unwired: 4 in, 5 out]
        }
      }
    }
    frame #3 {
      n192 = local read "connection reference"() -> (w279:T2)
      n193 = call <vilib>:"DB Tools Close Connection.vi"("connection reference"=w279) -> ("error out"=w277:errorcluster)  [unwired: 6 in]
      n194 = control-ref of="This VI"() -> (w278:refnum<vi>)
      n195 = invoke class="VI" method="FP.Close"(reference=w278, error in=w277) -> ()  [unwired: 1 in, 3 out]
    }
  }
